vi "writeToXML.vi"(8 "error in (no error)":errorcluster, 10 "ClassLabel":string, 11 "Offset in":refnum<class "Offset.lvclass">) -> (0 "error out":errorcluster, 2 "XML out":string, 3 "Offset out":refnum<class "Offset.lvclass">)   [LabVIEW 2014, in "TCSDataDefinitions.lvlib" / "TCSCommand.lvlib" / "OffsetCommands.lvlib" / "Offset.lvclass"]
uses:
  Offset.lvclass
  Offset.lvclass/Offset.ctl
  TargetOffsetCommands/TargetOffsetCommands.lvclass
  OffsetDef/OffsetDef/OffsetDef.lvclass
  <userlib>/Common/XML/XMLGenerator/XMLGenerator.lvclass
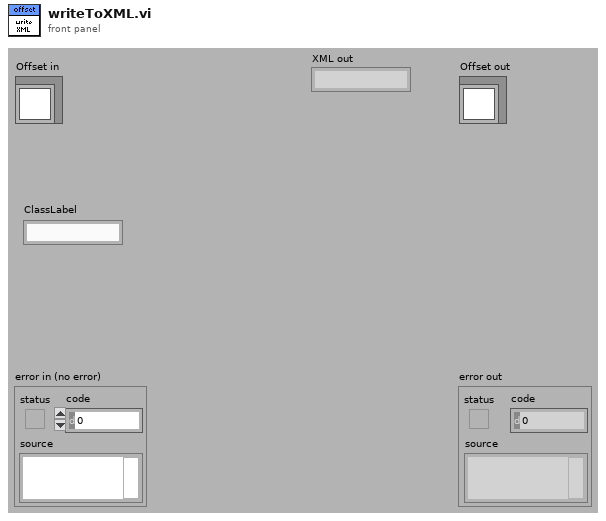
[diagram p1: front panel]
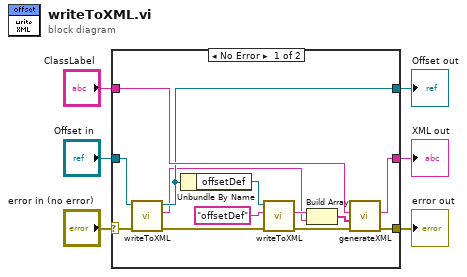
[diagram p0: block diagram]
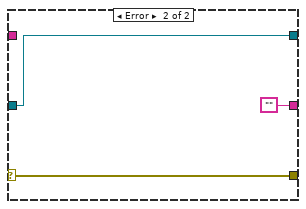
[diagram p2: hidden frame]
diagram:
  n1 = case shown="No Error" "error in (no error)" {
    selector: "error in (no error)" -> [w11 w22]
    tunnel: [w15 w22] -> w5
    tunnel: [w12 w21] -> w3
    tunnel: "Offset in" -> [w13 w21]
    tunnel: "ClassLabel" -> [w14 _]
    tunnel: [w7 ""] -> w1
    frame No Error {
      n2 = call-parent "writeToXML.vi"("error in (no error)"=w11, "TargetOffsetCommands in"=w13) -> ("error out"=w10:errorcluster, "XML out"=w8:string, "TargetOffsetCommands out"=w12:refnum<class "Offset.lvclass">)  [unwired: 7 in]
      n3 = Unbundle By Name(w12) -> ("offsetDef"=w19:refnum<class "OffsetDef.lvclass">)
      n4 = call-dynamic "writeToXML.vi"("error in (no error)"=w10, "ClassLabel"="offsetDef", "OffsetDef in"=w19) -> ("error out"=w16:errorcluster, "XML out"=w17:string)  [unwired: 6 in, 1 out]
      n5 = Build Array(w17, w8) -> (w18:string[])
      n6 = call <userlib>:"generateXML.vi"("error in"=w16, "childrenXML"=w18, "elementName"=w14) -> ("error out"=w15:errorcluster, "XML out"=w7:string)  [unwired: 6 in, 1 out]
    }
    frame Error {
    }
  }
  "error out" <- w5
  "Offset out" <- w3
  "XML out" <- w1
